vi "释放图像缓存.vi"(8 "错误输入（无错误）":errorcluster, 9 "灰度图像":T1, 11 "缓存数据":T2) -> (0 "错误输出":errorcluster)   [LabVIEW 2015]
uses:
  <vilib>/vision/Image Controls.llb/IMAQ Image.ctl
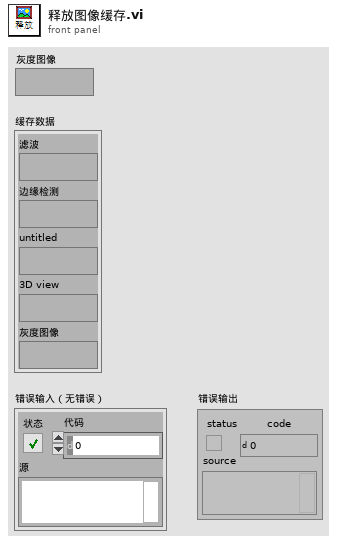
[diagram p1: front panel]
types:
  T1 = typedef "IMAQ Image.ctl" = refnum<image>
  T2 = cluster{"滤波":T1, "边缘检测":T1, "untitled":T1, "3D view":T1, "灰度图像":T1}
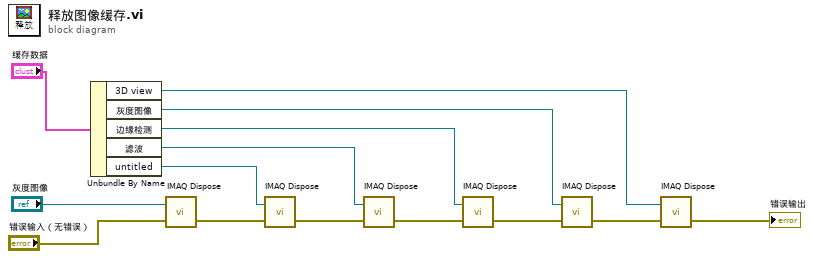
[diagram p0: block diagram]
diagram:
  n1 = Unbundle By Name("缓存数据") -> ("3D view"=w9:T1, "灰度图像"=w10:T1, "边缘检测"=w11:T1, "滤波"=w12:T1, "untitled"=w13:T1)
  n2 = call "IMAQ Dispose"("Image"="灰度图像", "error in (no error)"="错误输入（无错误）") -> ("error out"=w3:errorcluster)  [unwired: 4 in]
  n3 = call "IMAQ Dispose"("Image"=w13, "error in (no error)"=w3) -> ("error out"=w5:errorcluster)  [unwired: 4 in]
  n4 = call "IMAQ Dispose"("Image"=w12, "error in (no error)"=w5) -> ("error out"=w4:errorcluster)  [unwired: 4 in]
  n5 = call "IMAQ Dispose"("Image"=w11, "error in (no error)"=w4) -> ("error out"=w2:errorcluster)  [unwired: 4 in]
  n6 = call "IMAQ Dispose"("Image"=w10, "error in (no error)"=w2) -> ("error out"=w1:errorcluster)  [unwired: 4 in]
  n7 = call "IMAQ Dispose"("Image"=w9, "error in (no error)"=w1) -> ("error out"=→"错误输出":errorcluster)  [unwired: 4 in]
